vi "ApplyDeadband_Example.vi"() -> ()   [LabVIEW 2019]
uses:
  <vilib>/Rock Robotics/WPI/ThirdParty/JAS_Junk/TrajLib/Trajectory_Library.lvlib
panel:
  in  "Noise Magnitude":dbl=0.05
  in  "Use Noise":bool
  out "Output with\ndeadband applied":dbl format="%14.3f"
  in  "Deadband":dbl=0.2
  in  "Input":dbl(slide)=-0.015748031496062964 scale=-1.0..1.0
  out "Clamped Vlue":cluster{"Input":dbl, "Result":dbl}(graph)
  out "Raw Input":dbl=10.0 format="%14.3f"
  in  "Max Magnitude":dbl=1.0
  # "Analog  - ApplyDeadband - Example"
  # "Optional - Defaults to 1.0"
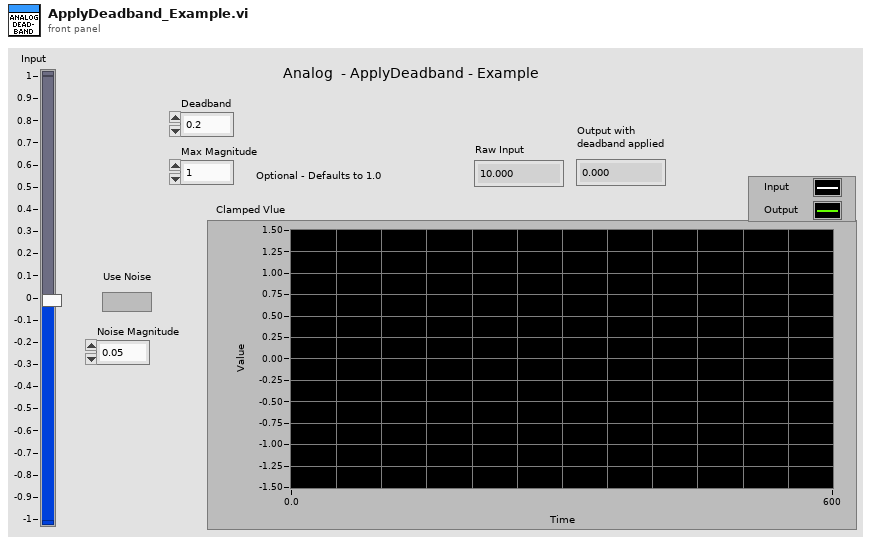
[diagram p1: front panel]
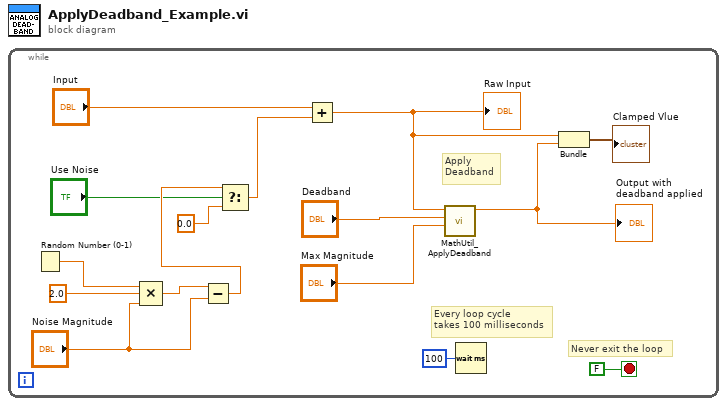
[diagram p0: block diagram]
diagram:
  n1 = while {
    stop <- FALSE stop-if-true
    # "Apply\nDeadband"
    # "Every loop cycle\ntakes 100 milliseconds"
    # "Never exit the loop"
    n2 = Random Number (0-1)() -> (number: 0 to 1=w10:dbl)
    n3 = Compound Arithmetic op=MULTIPLY(w10, 2.0 ("y"), "Noise Magnitude") -> (w8:dbl)
    n4 = Subtract(x=w8, y="Noise Magnitude") -> (x-y=w6:dbl)
    n5 = Select(t=w6, s="Use Noise", f=0.0) -> (s? t:f=w3:dbl)
    n6 = Add(x="Input", y=w3) -> (x+y=w1:dbl)
    "Raw Input" <- w1
    n7 = call <vilib>:"MathUtil_ApplyDeadband.vi"("Max Magnitude"="Max Magnitude", "Deadband"="Deadband", "Value"=w1) -> ("Result"=w13:dbl)  [unwired: 8 in]
    "Output with\ndeadband applied" <- w13
    n8 = Wait (ms)(milliseconds to wait=u32 100) -> ()  [unwired: 1 out]
    n9 = Bundle(w1, "Result"=w13) -> (→"Clamped Vlue":cluster{dbl, "Result":dbl})  [unwired: 1 in]
  }
